vi "NPC3SG Connect v10.6.1.vi"(4 "Drive Port":refnum<visa-resource-name>="COM5" caption="Visa Port") -> (0 "Success":bool, 1 "Drive Visa Name":refnum<visa-resource-name>)   [LabVIEW 2010]
uses:
  drivers/Newport NPC3SG/SubNPC3SG.llb/device variables.vi
panel:
  out "Read Error":errorcluster caption="error out" {"code" format="%x"}
  out "Connection Error":errorcluster
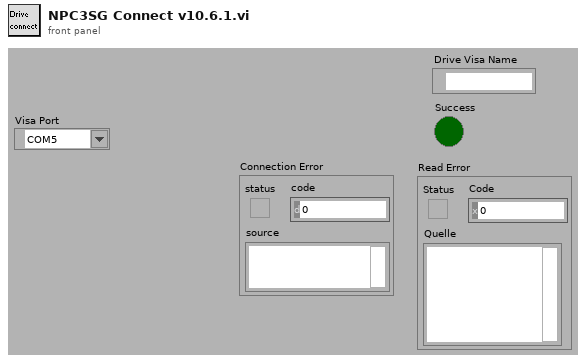
[diagram p1: front panel]
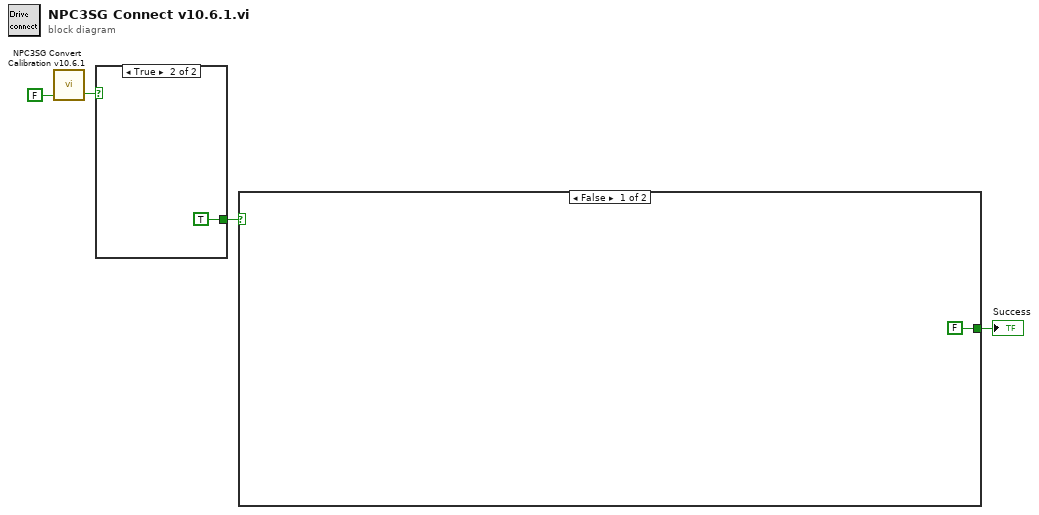
[diagram p0: block diagram]
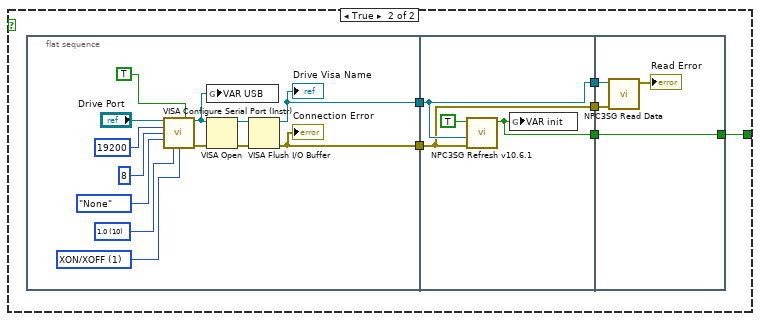
[diagram p2: hidden frame]
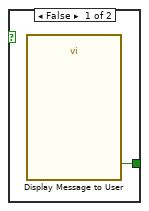
[diagram p3: hidden frame]
diagram:
  n1 = call "NPC3SG Convert Calibration v10.6.1.vi"("Is Voltage?"=FALSE) -> ("Has calibration?"=w3:bool)  [unwired: 2 in, 1 out]
  n2 = case shown="True" w3 {
    tunnel: [w5 TRUE ("OK")] -> w1
    frame False {
      n3 = call "Display Message to User"() -> ("OK"=w5:bool)  [unwired: 10 in, 1 out]
    }
    frame True {
    }
  }
  n4 = case shown="False" w1 {
    tunnel: [FALSE ("init ok??") w8] -> w2
    frame False {
    }
    frame True {
      n5 = flat-sequence {
        tunnel: [w16] -> w13
        tunnel: [w15] -> w12
        tunnel: w13 -> [w29]
        tunnel: w12 -> [w28]
        tunnel: [w29] -> w11
        tunnel: [w28] -> w10
        tunnel: [w27] -> w9
        tunnel: w11 -> [w33]
        tunnel: w10 -> [w32]
        tunnel: [w31] -> w8
        tunnel: w9 -> [w31]
        frame #0 {
          w18 = u16 1 items=["Kein", "XON/XOFF", "RTS/CTS", "XON/XOFF & RTS/CTS", "DTR/DSR", "XON/XOFF & DTR/DSR"] ("flow control (0:none)")
          w26 = u16 10 items=["1.0"=10, "1.5"=15, "2.0"=20] ("stop bits (10: 1 bit)")
          n6 = call <vilib>:"VISA Configure Serial Port (Instr).vi"("VISA resource name"="Drive Port", "Enable Termination\nChar (T)"=TRUE ("Enable Termination\nChar (T)"), "baud rate (9600)"=u32 19200, "data bits (8)"=u16 8, "parity (0:none)"=enum16{"None", "Odd", "Even", "Mark", "Space"}."None", "stop bits (10: 1 bit)"=w26, "flow control (0:none)"=w18) -> ("VISA resource name out"=w17:refnum<visa-resource-name>, "error out"=w20:errorcluster)  [unwired: 7 in]
          n7 = global write "device variables.vi" "VAR USB"(w17) -> ()
          n8 = VISA Open(error in (no error)=w20, VISA resource name=w17) -> (VISA resource name=w21:refnum<visa-resource-name>, error out=w22:errorcluster)  [unwired: 3 in]
          n9 = VISA Flush I/O Buffer(VISA resource name=w21, error in (no error)=w22) -> (VISA resource name out=w16:refnum<visa-resource-name>, error out=w15:errorcluster)  [unwired: 1 in]
          "Connection Error" <- w15
          "Drive Visa Name" <- w16
        }
        frame #1 {
          n10 = call "NPC3SG Refresh v10.6.1.vi"("error in"=w28, "VISA-Ressourcen-Name (In)"=w29, "reset all"=TRUE) -> ("init ok??"=w27:bool)  [unwired: 8 in]
          n11 = global write "device variables.vi" "VAR init"(w27) -> ()
        }
        frame #2 {
          n12 = call "NPC3SG Read Data.vi"("VISA resource name in"=w33, "error in"=w32) -> ("error ende"=→"Read Error":errorcluster)  [unwired: 8 in]
        }
      }
    }
  }
  "Success" <- w2
